vi "Spec_GUI.vi"(10 "stop 2":refnum<vi>, 11 "GUI_cluster":T1={"Sub Panel"=refnum, "GUIdevice"="Bella_LP_Mode", "CtlRef"=refnum, "User Event in"=refnum}) -> ()   [LabVIEW 2013]
uses:
  Shared/GUI_Template/GUI_master/tcp new data cluster.ctl
  Controls/eventtypdef1.ctl
  Shared/GUI_Template/GUI_master/tcp_new_data_event.ctl
  Controls/GUI_cluster.ctl
panel:
  in  "stop":bool
  in  "save::1":bool caption="save"
  in  "trigger::1":bool caption="trigger"
  out "counts::1":dbl[](array[numeric])
  out "wavelength::1":dbl[](array[numeric])
  out "spec":cluster{"counts":dbl[], "wavelength":dbl[]}(graph)
  out "tcp data event":T2
  out "GUIdevice 1":string="StagingHexapodPI"
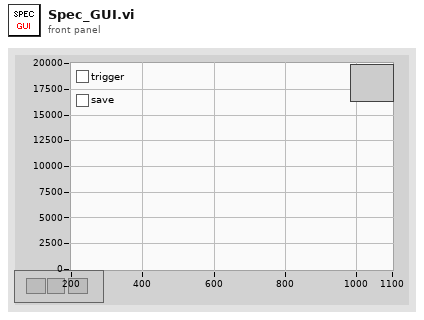
[diagram p1: front panel]
types:
  T1 = typedef "GUI_cluster.ctl" = cluster{"Sub Panel":refnum<vi>, "GUIdevice":string, "CtlRef":refnum<vi>, "User Event in":refnum<user-event>}
  T2 = typedef "tcp_new_data_event.ctl" = refnum<user-event>
  T3 = typedef "eventtypdef1.ctl" = cluster{"label":string, "Sub Panel":refnum<vi>, "CtlRef":refnum<vi>, "This VI":refnum<vi>}
  T4 = typedef "tcp new data cluster.ctl" = cluster{"EventEnum":enum16{"new data", "connection status update"}, "Device name":string}
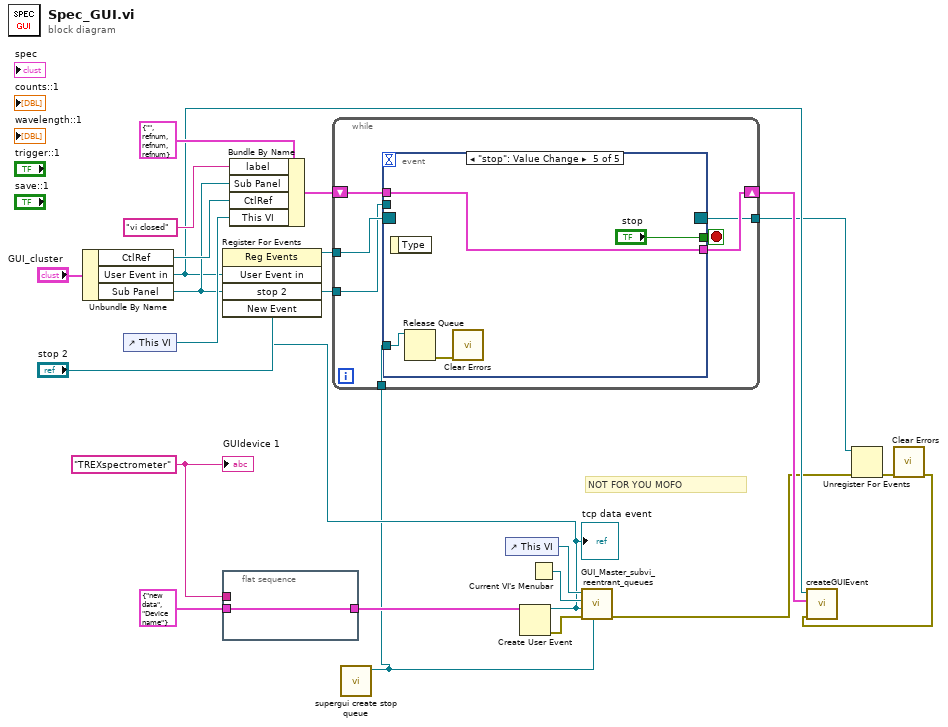
[diagram p0: block diagram]
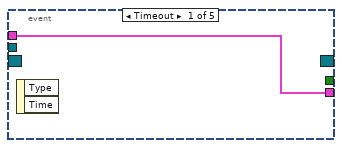
[diagram p2: hidden frame]
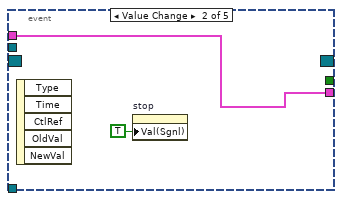
[diagram p3: hidden frame]
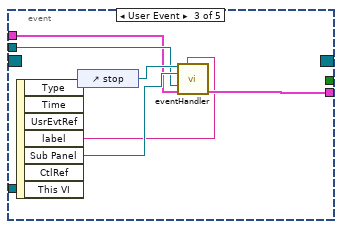
[diagram p4: hidden frame]
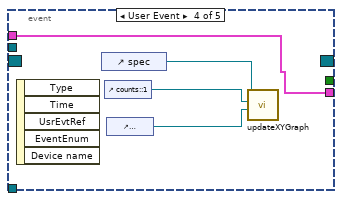
[diagram p5: hidden frame]
diagram:
  w14 = "TREXspectrometer" ("GUIdevice")
  # "NOT FOR YOU MOFO"
  n1 = Unbundle By Name("GUI_cluster") -> ("CtlRef"=w16:refnum<vi>, "User Event in"=w9:refnum<user-event>, "Sub Panel"=w11:refnum<vi>)
  n2 = control-ref of="This VI"() -> (w15:refnum<vi>)
  n3 = flat-sequence {
    tunnel: T4 {"EventEnum"=enum."new data", "Device name"="Device name"} ("New Event") -> [w24]
    tunnel: [w24] -> w17
    tunnel: w14 -> [_]
    frame #0 {
    }
  }
  n4 = Bundle By Name(cluster=T3 {"label"="", "Sub Panel"=refnum, "CtlRef"=refnum, "This VI"=refnum} ("event data"), "label"="vi closed", "Sub Panel"=w11, "CtlRef"=w16, "This VI"=w15) -> (w10:T3)
  n5 = call "supergui create stop queue.vi"() -> ("STOP Queue out"=w1:refnum<queue>)  [unwired: 11 in]
  n6 = control-ref of="This VI"() -> (w23:refnum<vi>)
  n7 = Create User Event(user event datatype=w17) -> (user event=w6:refnum<user-event>, error out=w21:errorcluster)  [unwired: 1 in]
  "tcp data event" <- w6
  n8 = register-events(w9, "stop 2", w6) -> (reference out=w13:refnum<event-registration>)  [unwired: 2 in, 1 out]
  n9 = while {
    tunnel: w13 -> [w31]
    tunnel: w11 -> [w29]
    shift-right: [w27] -> w8
    shift-left: w10 -> [w28]
    tunnel: [w26] -> w4
    tunnel: w1 -> [w25]
    stop <- w30 stop-if-true
    n10 = event shown="[4] \"stop\": Value Change" {
      selector: w31 -> [_ _ _ _ _]
      dyn-events: [_ _ _ _ _] -> w26
      timeout: _ -> [_ _ _ _ _]
      tunnel: [_ _ _ _ "stop"] -> w30
      tunnel: w29 -> [_ _ w38 _ _]
      tunnel: w28 -> [w32 w34 w37 w41 w47]
      tunnel: [w32 w34 w36 w41 w47] -> w27
      tunnel: w25 -> [_ _ _ _ w46]
      event Timeout {
        n11 = event-data() -> ()  [unwired: 1 in, 2 out]
      }
      event Value Change {
        n12 = event-data() -> ()  [unwired: 1 in, 5 out]
        n13 = property on="stop" class="Bool (strict)"("Val(Sgnl)"=TRUE ("Value (Signaling)")) -> ()  [unwired: 2 in, 2 out]
      }
      event User Event {
        n14 = event-data() -> ("label"=w35:string, "Sub Panel"=w39:refnum<vi>)  [unwired: 1 in, 5 out]
        n15 = control-ref of="stop"() -> (w40:refnum<vi>)
        n16 = call "eventHandler.vi"("Boolean in"=w40, "label"=w35, "Sub Panel 2"=w39, "Sub Panel"=w38, "event data in"=w37) -> ("event data out"=w36:T3)  [unwired: 10 in]
      }
      event User Event {
        n17 = event-data() -> ()  [unwired: 1 in, 5 out]
        n18 = control-ref of="spec"() -> (w42:refnum<vi>)
        n19 = control-ref of="counts::1"() -> (w44:refnum<vi>)
        n20 = control-ref of="wavelength::1"() -> (w43:refnum<vi>)
        n21 = call "updateXYGraph.vi"("wavelength"=w43, "counts"=w44, "XYGraph in"=w42) -> ()  [unwired: 7 in, 2 out]
      }
      event "stop": Value Change {
        n22 = event-data() -> ()  [unwired: 1 in, 1 out]
        n23 = Release Queue(queue=w46) -> (error out=w45:errorcluster)  [unwired: 2 in, 2 out]
        n24 = call <vilib>:"Clear Errors.vi"("error in (no error)"=w45) -> ()  [unwired: 6 in, 1 out]
      }
    }
  }
  n25 = Current VI's Menubar() -> (w22:refnum<k9>)
  n26 = call "GUI_Master_subvi_reentrant_queues.vi"("STOP Queue in"=w1, "error in (no error)"=w21, "tcp data event"=w6, "Caller menu reference"=w22, "Caller VI ref"=w23) -> ("error out"=w3:errorcluster)  [unwired: 6 in]
  n27 = Unregister For Events(event registration refnum=w4, error in=w3) -> (error out=w5:errorcluster)
  n28 = call <vilib>:"Clear Errors.vi"("error in (no error)"=w5) -> ("error out"=w2:errorcluster)  [unwired: 6 in]
  n29 = call "createGUIEvent.vi"("error in (no error)"=w2, "event data"=w8, "User Event in"=w9) -> ()  [unwired: 8 in, 1 out]
  "GUIdevice 1" <- w14
